vi "AI Configure Channel's.vi"(8 "error in (no error)":errorcluster, 11 "Data Cluster in":T2 {"AI Config Data"."Analog Input Timing"."sample mode" items=["Finite Samples"=10178, "Continuous Samples"=10123, "Hardware Timed Single Point"=12522]}) -> (0 "error out":errorcluster, 3 "Data Cluster out":T2 {"AI Config Data"."Analog Input Timing"."sample mode" items=["Finite Samples"=10178, "Continuous Samples"=10123, "Hardware Timed Single Point"=12522]}, 7 "Configuration Data":T3[](array[typedef]))   [LabVIEW 2024]
uses:
  Analog Output/Controls/AO Channel Configuration Cluster.ctl
  Controls/Analog Input SM Data Cluster.ctl
  Analog Output/Controls/AIO Command Q Cluster.ctl
  Analog Output/Controls/AO Interface Data Cluster.ctl
  Analog Output/Controls/AO Timing Cluster.ctl
  Main Engine/Controls/Main Engine JSON Command State.ctl
  TCP Engine/Controls/TCP Engine I&O  Interupt Cluster.ctl
  Host-DQMH/Configuration/Analog Input Single Channel Data--Cluster.ctl
  Host-DQMH/Configuration/Config-Channel Type.ctl
  Host-DQMH/Configuration/Channel Sub-Type.ctl
  Main Engine/Controls/Main Engine Config Confirmation Cluster.ctl
  Host-DQMH/Configuration/AI-Voltage Channel Data's.ctl
  Host-DQMH/Configuration/AI-Current Channel Data's--Cluster.ctl
  Host-DQMH/Configuration/AI-Thermocouple Data's.ctl
  <vilib>/DAQmx/create/channels.llb/DAQmx Create Channel (AI-Voltage-Basic).vi
  <vilib>/DAQmx/create/channels.llb/DAQmx Create Channel (AI-Current-Basic).vi
  <vilib>/DAQmx/create/channels.llb/DAQmx Create Channel (AI-Temperature-Thermocouple).vi
  <vilib>/DAQmx/configure/timing.llb/DAQmx Timing (Sample Clock).vi
  Host-DQMH/Configuration/Configuration.lvlib
  TCP Engine/TCP Engine.lvlib
panel:
  out "AI Configuration.Analog Input Timing":T1={"samples per channel"=1000, "sample mode"=10178, "Sampling Rate"=1000.0} {"sample mode" items=["Finite Samples"=10178, "Continuous Samples"=10123, "Hardware Timed Single Point"=12522]}
  out "Configured Channel's":string[](array[string])
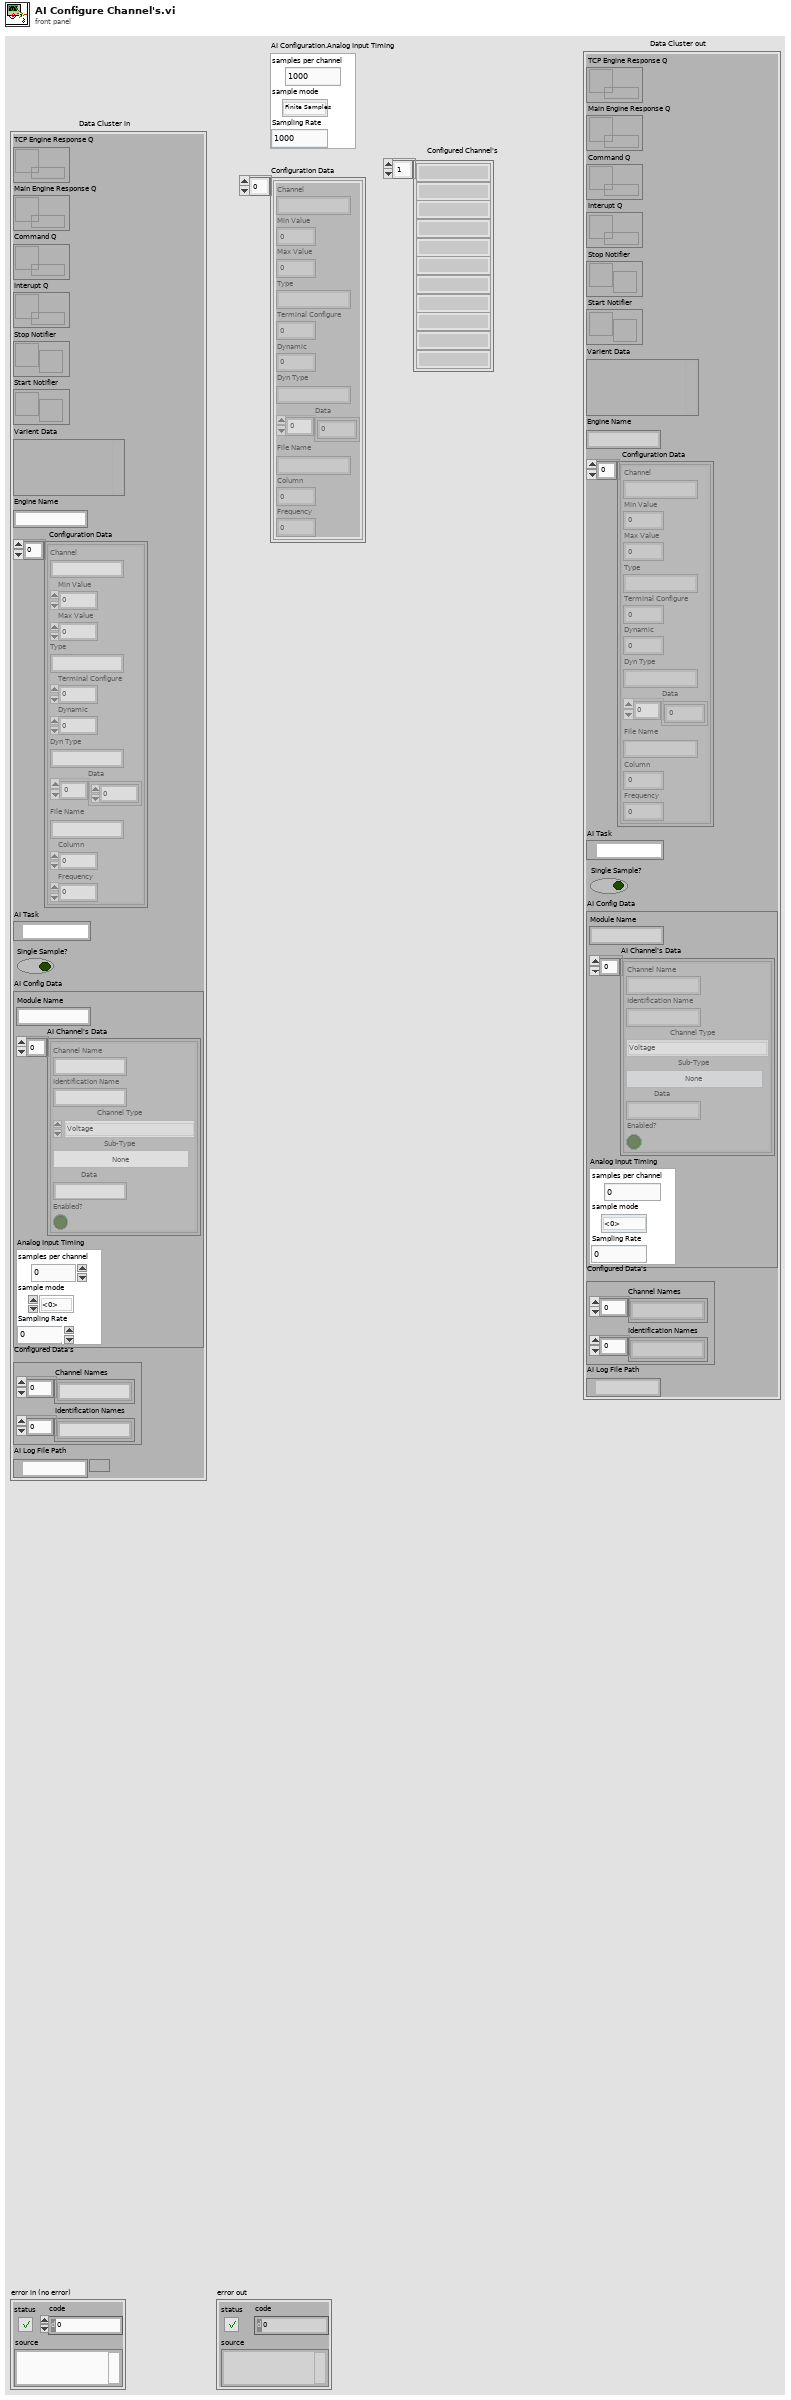
[diagram p1: front panel]
types:
  T1 = typedef "AO Timing Cluster.ctl" = cluster{"samples per channel":i32, "sample mode":i32, "Sampling Rate":dbl}
  T2 = typedef "Analog Input SM Data Cluster.ctl" = cluster{"TCP Engine Response Q":refnum<queue>, "Main Engine Response Q":refnum<queue>, "Command Q":refnum<queue>, "Interupt Q":refnum<queue>, "Stop Notifier":refnum<notifier>, "Start Notifier":refnum<notifier>, "Varient Data":variant, "Engine Name":string, "Configuration Data":T3[], "AI Task":refnum<k21>, "Single Sample?":bool, "AI Config Data":cluster{"Module Name":string, "AI Channel's Data":T4[], "Analog Input Timing":T1}, "Configured Data's":cluster{"Channel Names":string[], "Identification Names":string[]}, "AI Log File Path":path}
  T3 = typedef "AO Channel Configuration Cluster.ctl" = cluster{"Channel":string, "Min Value":dbl, "Max Value":dbl, "Type":string, "Terminal Configure":u16, "Dynamic":u8, "Dyn Type":string, "Data":dbl[], "File Name":string, "Column":i32, "Frequency":dbl}
  T4 = typedef "Configuration.lvlib/Analog Input Single Channel Data--Cluster.ctl" = cluster{"Channel Name":string, "Identification Name":string, "Channel Type":T5, "Sub-Type":T6, "Data":string, "Enabled?":bool}
  T5 = typedef "Configuration.lvlib/Config-Channel Type.ctl" = enum16{"Voltage", "Current", "Thermocouple", "Acclerometer"}
  T6 = typedef "Configuration.lvlib/Channel Sub-Type.ctl" = enum16{"None", "Pressure", "Force"}
  T7 = typedef "Main Engine Config Confirmation Cluster.ctl" = cluster{"Command":string, "Interface":string, "Status":string, "Board":string}
  T8 = typedef "Configuration.lvlib/AI-Voltage Channel Data's.ctl" = cluster{"input terminal configuration":i32, "maximum value":dbl, "minimum value":dbl, "units":i32}
  T9 = typedef "Configuration.lvlib/AI-Current Channel Data's--Cluster.ctl" = cluster{"maximum value":dbl, "minimum value":dbl, "input terminal configuration":i32, "external shunt resistor value":dbl, "units":i32, "shunt resistor location":i32}
  T10 = typedef "Configuration.lvlib/AI-Thermocouple Data's.ctl" = cluster{"thermocouple type":i32, "maximum value":dbl, "minimum value":dbl, "units":i32}
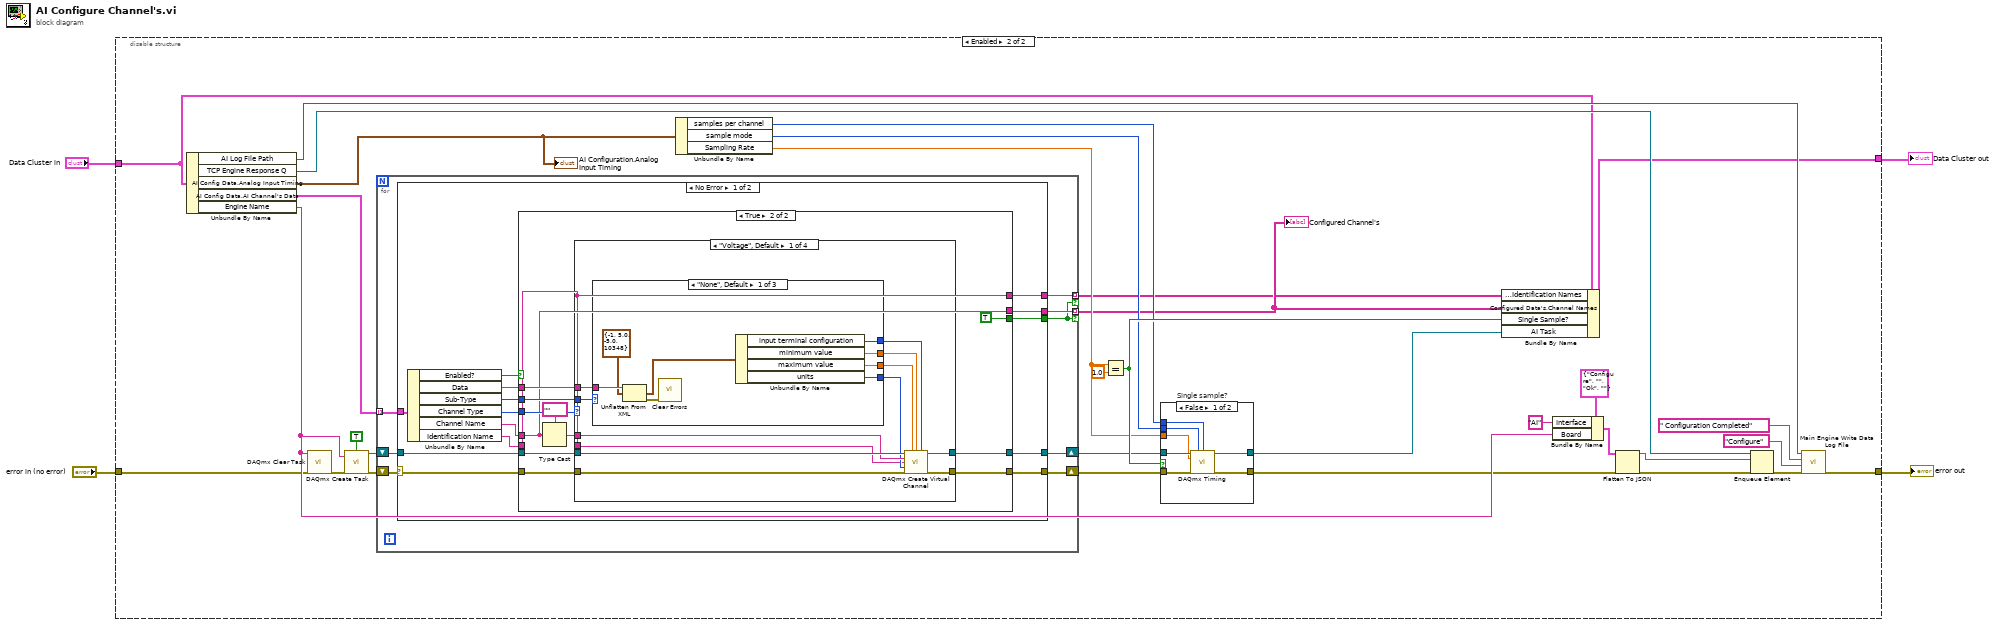
[diagram p0: block diagram]
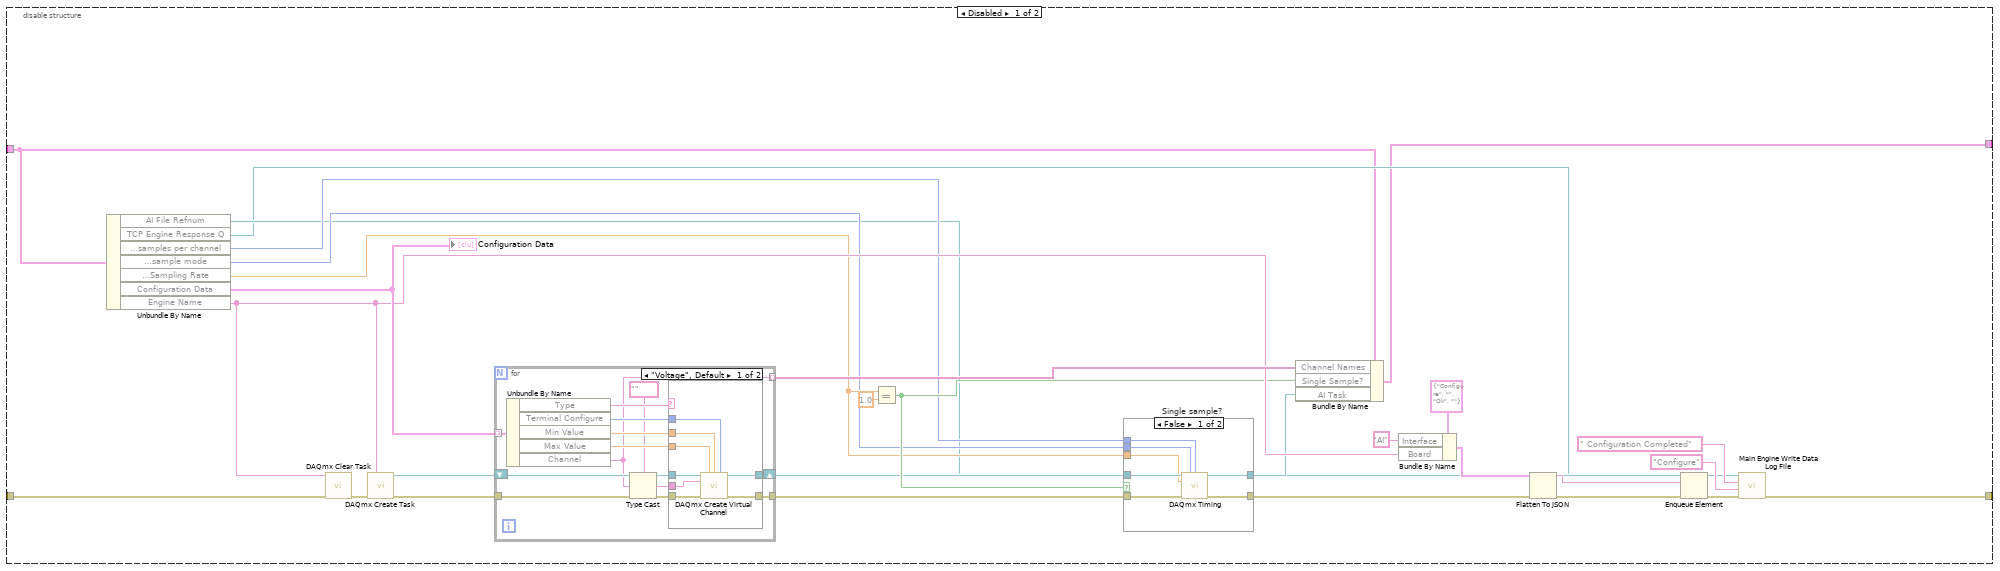
[diagram p2: hidden frame]
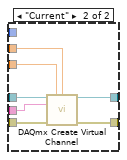
[diagram p4: hidden frame]
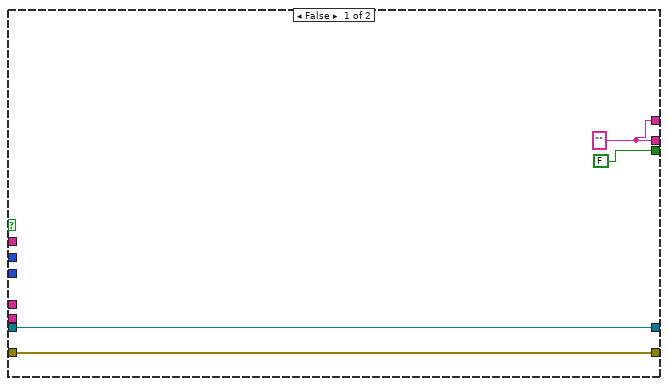
[diagram p6: hidden frame]
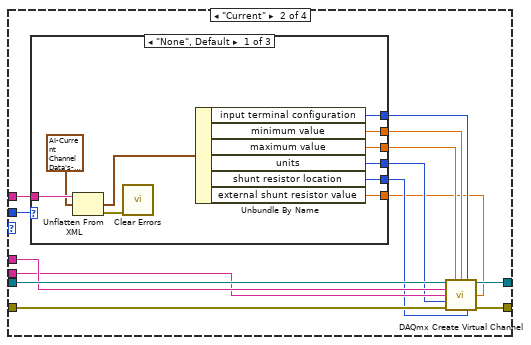
[diagram p9: hidden frame]
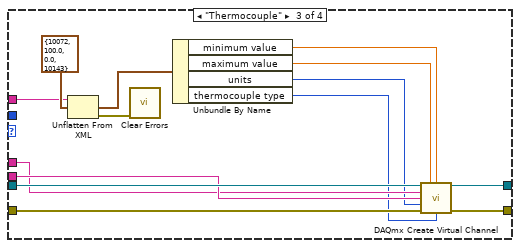
[diagram p12: hidden frame]
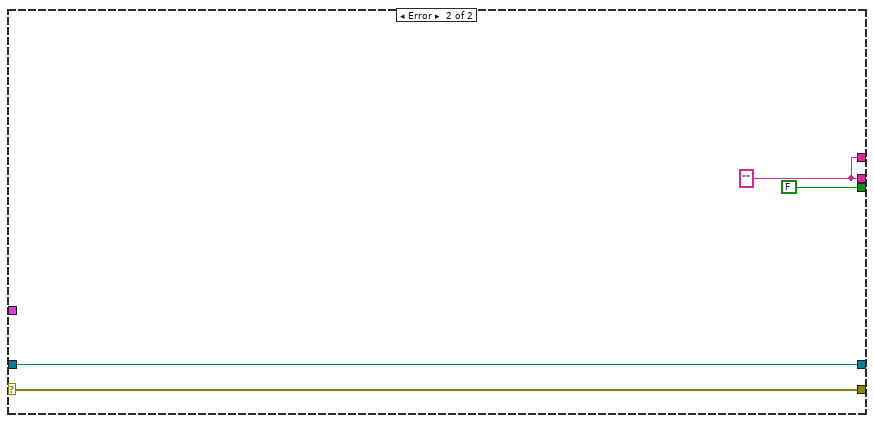
[diagram p14: hidden frame]
diagram:
  n1 = disable-structure shown="Enabled" {
    disable-tunnel: [w8 w79] -> w4
    disable-tunnel: "error in (no error)" -> [w7 w80]
    disable-tunnel: "Data Cluster in" -> [w6 w77]
    disable-tunnel: [w5 w78] -> w1
    frame Disabled {
      n2 = Unbundle By Name(w6) -> ("AI File Refnum"=w10:refnum<file>, "TCP Engine Response Q"=w9:refnum<queue>, "AI Config Data.Analog Input Timing.samples per channel"=w16:i32, "AI Config Data.Analog Input Timing.sample mode"=w17:i32, "AI Config Data.Analog Input Timing.Sampling Rate"=w20:dbl, "Configuration Data"=w33:T3[], "Engine Name"=w30:string)
      "Configuration Data" <- w33
      n3 = call <vilib>:"DAQmx Clear Task.vi"("task in"=w30, "error in"=w7) -> ("error out"=w11:errorcluster)  [unwired: 13 in]
      n4 = call <vilib>:"DAQmx Create Task.vi"("new task name"=w30, "error in"=w11) -> ("task out"=w13:refnum<k21>, "error out"=w12:errorcluster)  [unwired: 12 in]
      n5 = for {
        tunnel: w12 -> [w54]
        tunnel: [w53] -> w14
        tunnel: w33 -> [w50] mode=indexing
        tunnel: [w44] -> w31 mode=indexing
        shift-right: [w51] -> w15
        shift-left: w13 -> [w52]
        n6 = Unbundle By Name(w50) -> ("Type"=w47:string, "Terminal Configure"=w46:u16, "Min Value"=w49:dbl, "Max Value"=w48:dbl, "Channel"=w44:string)
        n7 = Type Cast(type=tag "" ("physical channels"), x=w44) -> (*(type *) &x=w43:tag)
        n8 = case shown="\"Voltage\", Default" w47 {
          tunnel: w54 -> [w62 w69]
          tunnel: [w61 w68] -> w53
          tunnel: w52 -> [w60 w67]
          tunnel: [w59 w66] -> w51
          tunnel: w49 -> [w58 w65]
          tunnel: w48 -> [w57 w64]
          tunnel: w46 -> [w56 _]
          tunnel: w43 -> [w55 w63]
          frame "Voltage", Default {
            n9 = call-poly <vilib>:"DAQmx Create Virtual Channel.vi"("task in"=w60, "maximum value"=w57, "minimum value"=w58, "input terminal configuration"=w56, "physical channels"=w55, "error in"=w62) -> ("task out"=w59:refnum<k21>, "error out"=w61:errorcluster)  [unwired: 8 in]
          }
          frame "Current" {
            n10 = call-poly <vilib>:"DAQmx Create Virtual Channel.vi"("task in"=w67, "maximum value"=w64, "minimum value"=w65, "physical channels"=w63, "error in"=w69) -> ("task out"=w66:refnum<k21>, "error out"=w68:errorcluster)  [unwired: 9 in]
          }
        }
      }
      n11 = Equal?(x=w20, y=1.0) -> (x = y?=w22:bool)
      n12 = case "Single sample?" shown="False" w22 {
        tunnel: w14 -> [w40 w41]
        tunnel: w15 -> [w39 w42]
        tunnel: [w38 w42] -> w21
        tunnel: w16 -> [w37 _]
        tunnel: w17 -> [w36 _]
        tunnel: w20 -> [w35 _]
        tunnel: [w34 w41] -> w23
        frame False {
          n13 = call-poly <vilib>:"DAQmx Timing.vi"("task/channels in"=w39, "sample mode"=w36, "samples per channel"=w37, "rate"=w35, "error in"=w40) -> ("task out"=w38:refnum<k21>, "error out"=w34:errorcluster)  [unwired: 9 in]
        }
        frame True {
        }
      }
      n14 = Bundle By Name(cluster=w6, "Channel Names"=w31, "Single Sample?"=w22, "AI Task"=w21) -> (w5:T2)
      n15 = Bundle By Name(cluster=T7 {"Command"="Configure", "Interface"="", "Status"="Ok", "Board"=""}, "Interface"="AI" ("SubCmd"), "Board"=w30) -> (w25:T7)
      n16 = Flatten To JSON(anything=w25, error in (no error)=w23) -> (JSON string=w28:string, 11:w26:errorcluster)  [unwired: 1 in]
      n17 = Enqueue Element(queue=w9, element=w28, error in (no error)=w26) -> (error out=w27:errorcluster)  [unwired: 1 in, 2 out]
      n18 = call "Main Engine Write Data Log File.vi"("error in"=w27, "State"="Configure", "Input Data"=" Configuration Completed", "Log file path In"=w10) -> ("error out"=w8:errorcluster)  [unwired: 6 in, 1 out]
    }
    frame Enabled {
      n19 = Unbundle By Name(w77) -> ("AI Log File Path"=w82:path, "TCP Engine Response Q"=w81:refnum<queue>, "AI Config Data.Analog Input Timing"=w71:T1, "AI Config Data.AI Channel's Data"=w101:T4[], "Engine Name"=w99:string)
      "AI Configuration.Analog Input Timing" <- w71
      n20 = call <vilib>:"DAQmx Clear Task.vi"("task in"=w99, "error in"=w80) -> ("error out"=w83:errorcluster)  [unwired: 13 in]
      n21 = call <vilib>:"DAQmx Create Task.vi"("new task name"=w99, "auto cleanup"=TRUE, "error in"=w83) -> ("task out"=w85:refnum<k21>, "error out"=w84:errorcluster)  [unwired: 11 in]
      n22 = for {
        tunnel: w101 -> [w114] mode=indexing
        tunnel: [w113] -> w72 mode=indexing if=w111
        shift-right: [w115] -> w87
        shift-left: w85 -> [w116]
        shift-right: [w117] -> w86
        shift-left: w84 -> [w118]
        tunnel: [w112] -> w70 mode=indexing if=w111
        n23 = case shown="No Error" w118 {
          selector: w118 -> [w132 w212]
          tunnel: [w131 w212] -> w117
          tunnel: w116 -> [w130 w211]
          tunnel: [w129 w211] -> w115
          tunnel: w114 -> [w128 _]
          tunnel: [w121 w209] -> w113
          tunnel: [w120 FALSE] -> w111
          tunnel: [w119 w209] -> w112
          frame No Error {
            n24 = Unbundle By Name(w128) -> ("Enabled?"=w122:bool, "Data"=w124:string, "Sub-Type"=w127:T6, "Channel Type"=w126:T5, "Channel Name"=w125:string, "Identification Name"=w123:string)
            n25 = case shown="True" w122 {
              tunnel: w132 -> [w135 w148]
              tunnel: [w135 w147] -> w131
              tunnel: w130 -> [w136 w146]
              tunnel: [w136 w145] -> w129
              tunnel: w127 -> [_ w144]
              tunnel: w126 -> [_ w143]
              tunnel: w125 -> [_ w139]
              tunnel: w124 -> [_ w140]
              tunnel: w123 -> [_ w137]
              tunnel: [w133 w139] -> w121
              tunnel: [FALSE TRUE] -> w120
              tunnel: [w133 w137] -> w119
              frame False {
                w133 = "" ("Channel Name")
              }
              frame True {
                n26 = Type Cast(type=tag "" ("physical channels"), x=w139) -> (*(type *) &x=w141:tag)
                n27 = case shown="\"Voltage\", Default" w143 {
                  tunnel: w148 -> [w160 w182 w206 w207]
                  tunnel: [w159 w181 w205 w207] -> w147
                  tunnel: w146 -> [w158 w180 w204 w208]
                  tunnel: [w157 w179 w203 w208] -> w145
                  tunnel: w141 -> [w156 w178 w201 _]
                  tunnel: w137 -> [w149 w176 w202 _]
                  tunnel: w144 -> [w155 w177 _ _]
                  tunnel: w140 -> [w154 w169 w195 _]
                  frame "Voltage", Default {
                    n28 = case shown="\"None\", Default" w155 {
                      tunnel: w154 -> [w164 _ _]
                      tunnel: [w168 _ _] -> w153
                      tunnel: [w167 _ _] -> w152
                      tunnel: [w166 _ _] -> w151
                      tunnel: [w165 _ _] -> w150
                      frame "None", Default {
                        n29 = Unflatten From XML(xml string=w164, type=T8 {"input terminal configuration"=-1, "maximum value"=5.0, "minimum value"=-5.0, "units"=10348} ("AI-Voltage Data's")) -> (value=w162:T8, error out=w161:errorcluster)  [unwired: 1 in]
                        n30 = call <vilib>:"Clear Errors.vi"("error in (no error)"=w161) -> ()  [unwired: 5 in, 2 out]
                        n31 = Unbundle By Name(w162) -> ("input terminal configuration"=w168:i32, "minimum value"=w167:dbl, "maximum value"=w166:dbl, "units"=w165:i32)
                      }
                      frame "Pressure" {
                      }
                      frame "Force" {
                      }
                    }
                    n32 = call-poly <vilib>:"DAQmx Create Virtual Channel.vi"("task in"=w158, "maximum value"=w151, "minimum value"=w152, "input terminal configuration"=w153, "physical channels"=w156, "name to assign"=w149, "units"=w150, "error in"=w160) -> ("task out"=w157:refnum<k21>, "error out"=w159:errorcluster)  [unwired: 6 in]
                  }
                  frame "Current" {
                    n33 = case shown="\"None\", Default" w177 {
                      tunnel: [w192 _ _] -> w175
                      tunnel: [w191 _ _] -> w174
                      tunnel: [w190 _ _] -> w173
                      tunnel: [w189 _ _] -> w172
                      tunnel: [w188 _ _] -> w171
                      tunnel: [w187 _ _] -> w170
                      tunnel: w169 -> [w184 _ _]
                      frame "None", Default {
                        n34 = Unflatten From XML(xml string=w184, type=T9 {"maximum value"=1.01, "minimum value"=-0.01, "input terminal configuration"=-1, "external shunt resistor value"=249.0, "units"=10342, "shunt resistor location"=-1} ("AI-Current")) -> (value=w186:T9, error out=w185:errorcluster)  [unwired: 1 in]
                        n35 = call <vilib>:"Clear Errors.vi"("error in (no error)"=w185) -> ()  [unwired: 5 in, 2 out]
                        n36 = Unbundle By Name(w186) -> ("input terminal configuration"=w192:i32, "minimum value"=w191:dbl, "maximum value"=w190:dbl, "units"=w189:i32, "shunt resistor location"=w188:i32, "external shunt resistor value"=w187:dbl)
                      }
                      frame "Pressure" {
                      }
                      frame "Force" {
                      }
                    }
                    n37 = call-poly <vilib>:"DAQmx Create Virtual Channel.vi"("task in"=w180, "maximum value"=w173, "minimum value"=w174, "input terminal configuration"=w175, "physical channels"=w178, "name to assign"=w176, "external shunt resistor value"=w170, "units"=w172, "error in"=w182, "shunt resistor location"=w171) -> ("task out"=w179:refnum<k21>, "error out"=w181:errorcluster)  [unwired: 4 in]
                  }
                  frame "Thermocouple" {
                    n38 = Unflatten From XML(xml string=w195, type=T10 {"thermocouple type"=10072, "maximum value"=100.0, "minimum value"=0.0, "units"=10143} ("AI-ThermoCouple")) -> (value=w194:T10, error out=w193:errorcluster)  [unwired: 1 in]
                    n39 = call <vilib>:"Clear Errors.vi"("error in (no error)"=w193) -> ()  [unwired: 5 in, 2 out]
                    n40 = Unbundle By Name(w194) -> ("minimum value"=w198:dbl, "maximum value"=w199:dbl, "units"=w200:i32, "thermocouple type"=w197:i32)
                    n41 = call-poly <vilib>:"DAQmx Create Virtual Channel.vi"("task in"=w204, "maximum value"=w199, "minimum value"=w198, "physical channels"=w201, "name to assign"=w202, "units"=w200, "error in"=w206, "thermocouple type"=w197) -> ("task out"=w203:refnum<k21>, "error out"=w205:errorcluster)  [unwired: 6 in]
                  }
                  frame "Acclerometer" {
                  }
                }
              }
            }
          }
          frame Error {
            w209 = "" ("Channel Name")
          }
        }
      }
      "Configured Channel's" <- w72
      n42 = Unbundle By Name(w71) -> ("samples per channel"=w74:i32, "sample mode"=w75:i32, "Sampling Rate"=w76:dbl)
      n43 = Equal?(x=w76, y=1.0) -> (x = y?=w91:bool)
      n44 = case "Single sample?" shown="False" w91 {
        tunnel: w86 -> [w108 w109]
        tunnel: w87 -> [w107 w110]
        tunnel: [w102 w110] -> w90
        tunnel: w74 -> [w106 _]
        tunnel: w75 -> [w105 _]
        tunnel: w76 -> [w104 _]
        tunnel: [w103 w109] -> w92
        frame False {
          n45 = call-poly <vilib>:"DAQmx Timing.vi"("task/channels in"=w107, "sample mode"=w105, "samples per channel"=w106, "rate"=w104, "error in"=w108) -> ("task out"=w102:refnum<k21>, "error out"=w103:errorcluster)  [unwired: 9 in]
        }
        frame True {
        }
      }
      n46 = Bundle By Name(cluster=w77, "Configured Data's.Identification Names"=w70, "Configured Data's.Channel Names"=w72, "Single Sample?"=w91, "AI Task"=w90) -> (w78:T2)
      n47 = Bundle By Name(cluster=T7 {"Command"="Configure", "Interface"="", "Status"="Ok", "Board"=""}, "Interface"="AI" ("SubCmd"), "Board"=w99) -> (w94:T7)
      n48 = Flatten To JSON(anything=w94, error in (no error)=w92) -> (JSON string=w97:string, 11:w95:errorcluster)  [unwired: 1 in]
      n49 = Enqueue Element(queue=w81, element=w97, error in (no error)=w95) -> (error out=w96:errorcluster)  [unwired: 1 in, 2 out]
      n50 = call "Main Engine Write Data Log File.vi"("error in"=w96, "State"="Configure", "Input Data"=" Configuration Completed", "Log file path In"=w82) -> ("error out"=w79:errorcluster)  [unwired: 6 in, 1 out]
    }
  }
  "error out" <- w4
  "Data Cluster out" <- w1
